vi "Enqueue Multiple.vi"(6 "In Front? (F)":bool, 8 "error in (no error)":errorcluster, 9 "Enqueue? (T)":bool=TRUE, 10 "Array":string[](array[string]), 11 "Queue in":refnum<queue>) -> (0 "error out":errorcluster, 3 "Queue out":refnum<queue>)   [LabVIEW 2017]
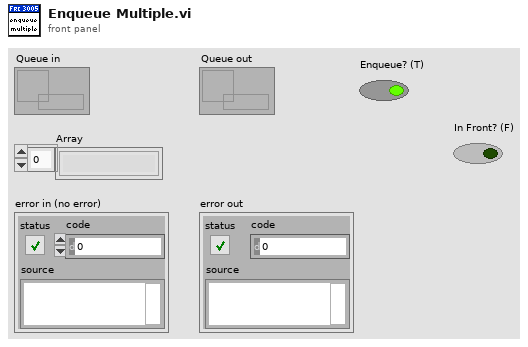
[diagram p1: front panel]
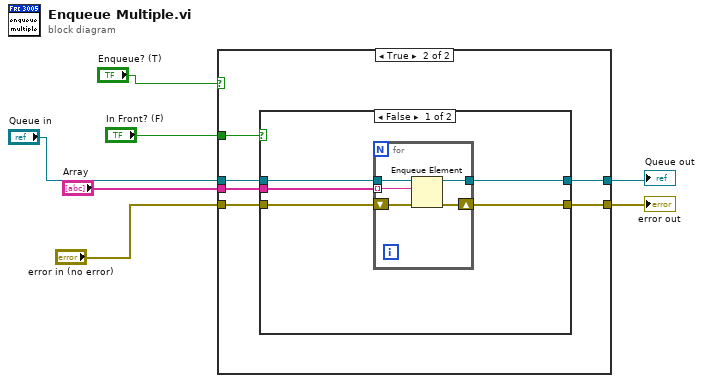
[diagram p0: block diagram]
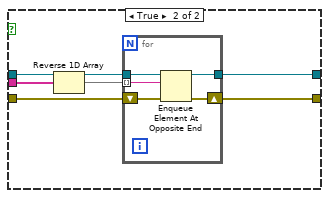
[diagram p3: hidden frame]
diagram:
  n1 = case shown="True" "Enqueue? (T)" {
    tunnel: [w9 w15] -> w7
    tunnel: [w8 w14] -> w6
    tunnel: "error in (no error)" -> [w8 w13]
    tunnel: "Queue in" -> [w9 w12]
    tunnel: "Array" -> [_ w11]
    tunnel: "In Front? (F)" -> [_ w10]
    frame False {
    }
    frame True {
      n2 = case shown="False" w10 {
        tunnel: [w20 w31] -> w15
        tunnel: [w19 w30] -> w14
        tunnel: w13 -> [w18 w29]
        tunnel: w12 -> [w17 w28]
        tunnel: w11 -> [w16 w27]
        frame False {
          n3 = for {
            tunnel: w16 -> [w25] mode=indexing
            shift-right: [w24] -> w19
            shift-left: w18 -> [w23]
            tunnel: [w22] -> w20
            tunnel: w17 -> [w21]
            n4 = Enqueue Element(queue=w21, element=w25, error in (no error)=w23) -> (queue out=w22:refnum<queue>, error out=w24:errorcluster)  [unwired: 1 in, 1 out]
          }
        }
        frame True {
          n5 = Reverse 1D Array(array=w27) -> (reversed array=w26:string[])
          n6 = for {
            tunnel: w26 -> [w36] mode=indexing
            shift-right: [w35] -> w30
            shift-left: w29 -> [w34]
            tunnel: [w33] -> w31
            tunnel: w28 -> [w32]
            n7 = Enqueue Element At Opposite End(queue=w32, element=w36, error in (no error)=w34) -> (queue out=w33:refnum<queue>, error out=w35:errorcluster)  [unwired: 1 in, 1 out]
          }
        }
      }
    }
  }
  "Queue out" <- w7
  "error out" <- w6
